vi "Write TX Port.vi"(0 "Refnum in":refnum<k20>, 2 "Timeout":i32=5000, 5 "TX Port":i32, 7 "Data":u8[](array[numeric]), 11 "error in (no error)":errorcluster) -> (4 "Refnum out":refnum<k20>, 15 "error out":errorcluster)   [LabVIEW 2020, in "My Network Host v1.lvlib"]
uses:
  My Network Host v1.lvlib
  Example Host Interface.ctl
  <vilib>/Utility/error.llb/Error Cluster From Error Code.vi
  <vilib>/rvi/errors/niLvFpgaAdjustHostInterfaceError.vi
  <vilib>/rvi/interface/nirviMethod/nirviMethod.xnode
  <vilib>/FPGAPlugInAG/Dynamic/niLvFpga_WriteFifo_Dynamic.vi
  <vilib>/rvi/errors/niLvFpgaMergeErrorWithErrorCode.vi
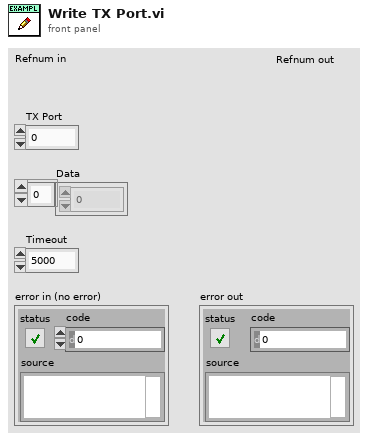
[diagram p1: front panel]
types:
  T1 = typedef "My Network Host v1.lvlib/Example Host Interface.ctl" = refnum<k20>
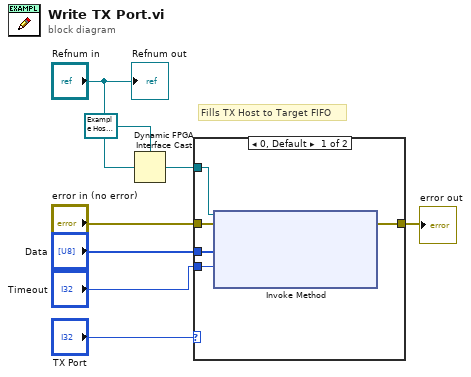
[diagram p0: block diagram]
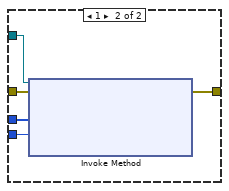
[diagram p2: hidden frame]
diagram:
  # "Fills TX Host to Target FIFO"
  n1 = Dynamic FPGA Interface Cast(Session In=T1 refnum ("Type"), Type="Refnum in") -> (Session Out=w2:T1)
  n2 = case shown="0, Default" "TX Port" {
    tunnel: w2 -> [w12 w18]
    tunnel: "error in (no error)" -> [w13 w17]
    tunnel: [w11 w16] -> w8
    tunnel: "Data" -> [w9 w15]
    tunnel: "Timeout" -> [w10 w14]
    frame 0, Default {
      n3 = xnode "Invoke Method"("FPGA VI Reference In"=w12, "error in"=w13, "Data"=w9, "Timeout (ms)"=w10) -> ("error out"=w11:errorcluster)  [unwired: 2 out]
    }
    frame 1 {
      n4 = xnode "Invoke Method"("FPGA VI Reference In"=w18, "error in"=w17, "Data"=w15, "Timeout (ms)"=w14) -> ("error out"=w16:errorcluster)  [unwired: 2 out]
    }
  }
  "error out" <- w8
  "Refnum out" <- "Refnum in"
